vi "SPADQ_MultiRecord.vi"(4 "Records":u32=1, 6 "Pts to Acquire":u32, 7 "ChanMask":u8(ring)=1 items=["A"=1, "B"=2, "A&B"=3], 8 "error in (no error)":errorcluster, 9 "adq_num":i32, 10 "adq_cu_ptr in":refnum<k24>, 11 "ADQAPI Ref":refnum<k24>) -> (0 "error out":errorcluster, 1 "RecordOut":T1={"Count"=1, "Presize"=1, "Length"=0}, 3 "ADQAPI Ref (out)":refnum<k24>)   [LabVIEW 2022 SP3]
doc: "_____AlazarTech, Scope_____\n\nSet the Trigger delay"
uses:
  C:/Windows/System32/ADQAPI_dotNet_helper.dll
  AlazarTech/-AlazarTools/Record.ctl
panel:
  out "ADQ_MultiRecordSetup":u32
  out "ADQ_MultiRecordSetChannelMask":u32
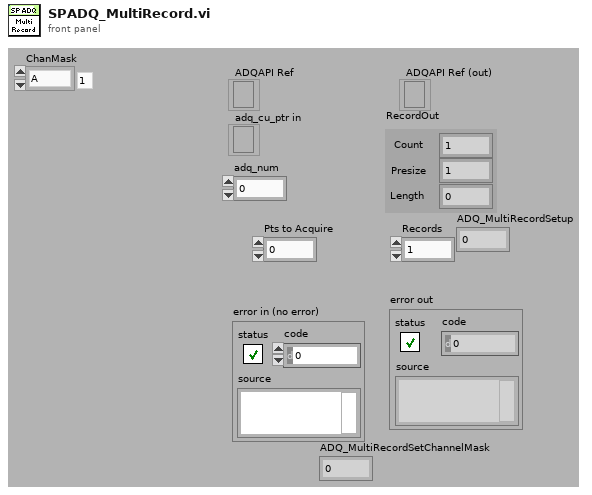
[diagram p1: front panel]
types:
  T1 = typedef "Record.ctl" = cluster{"Count":u32, "Presize":u32, "Length":u32}
  T2 = cluster{"Records":u32, "Count":u32, "Pts to Acquire":u32}
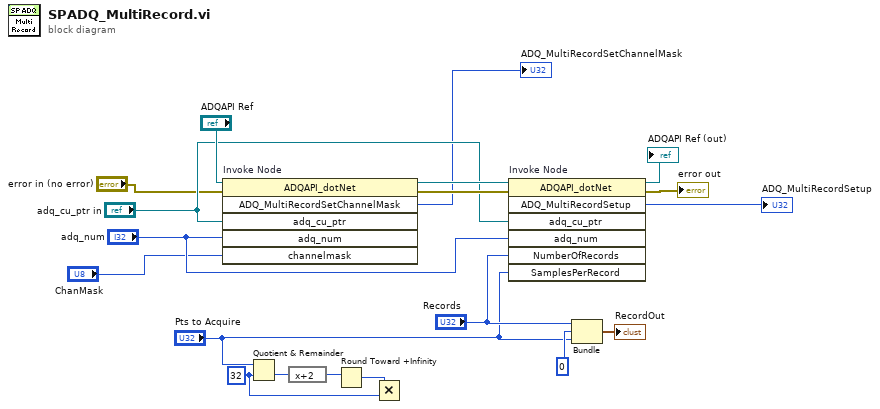
[diagram p0: block diagram]
diagram:
  w17 = u32 32 ("y")
  n1 = invoke on="Invoke Node" class="ADQAPI_dotNet" method="ADQ_MultiRecordSetChannelMask"(reference="ADQAPI Ref", error in="error in (no error)", "adq_cu_ptr"="adq_cu_ptr in", "adq_num"="adq_num", "channelmask"="ChanMask") -> (reference out=w8:refnum<k24>, error out=w7:errorcluster, "ADQ_MultiRecordSetChannelMask"=→"ADQ_MultiRecordSetChannelMask":u32)  [unwired: 1 in, 3 out]
  n2 = Quotient & Remainder(x="Pts to Acquire", y=w17) -> (floor(x/y)=w15:u32)  [unwired: 1 out]
  n3 = expression code="x+2"(w15) -> (w14:u32)
  n4 = Round Toward +Infinity(x=w14) -> (ceil(x): smallest int >= x=w16:u32)
  n5 = Multiply(x=w16, y=w17) -> ()  [unwired: 1 out]
  n6 = invoke on="Invoke Node" class="ADQAPI_dotNet" method="ADQ_MultiRecordSetup"(reference=w8, error in=w7, "adq_cu_ptr"="adq_cu_ptr in", "adq_num"="adq_num", "NumberOfRecords"="Records", "SamplesPerRecord"="Pts to Acquire") -> (reference out=→"ADQAPI Ref (out)":refnum<k24>, error out=→"error out":errorcluster, "ADQ_MultiRecordSetup"=→"ADQ_MultiRecordSetup":u32)  [unwired: 1 in, 4 out]
  n7 = Bundle("Records"="Records", "Count"=u32 0, "Pts to Acquire"="Pts to Acquire") -> (→"RecordOut":T2)  [unwired: 1 in]
